vi "Timer_ResetInternal.vi"(11 "in TIMER":T1 {"Accumulated TIme" format="%13.5p"; "StartTime" format="%13.5p"}) -> (3 "out TIMER":T1 {"Accumulated TIme" format="%13.5p"; "StartTime" format="%13.5p"})   [LabVIEW 2019, in "Trajectory_Library.lvlib"]
doc: "THIS IS AN INTERNAL ROUTINE. DO NOT USE.\n \nReset the timer by setting the time to 0. Make the timer startTime the current time so new requests will be relative now\n\nInputs:\n - Timer -- The Timer data cluster\n\nOutputs:\n - Timer -- The modified Timer data cluster"
uses:
  Trajectory_Library.lvlib
  TIMER.ctl
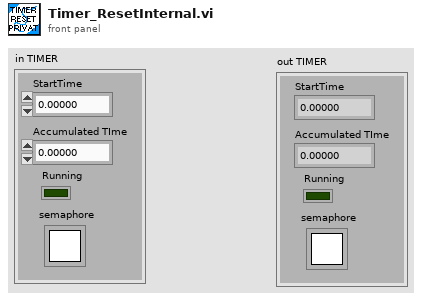
[diagram p1: front panel]
types:
  T1 = typedef "Trajectory_Library.lvlib/TIMER.ctl" = cluster{"StartTime":dbl, "Accumulated TIme":dbl, "Running":bool, "semaphore":T2}
  T2 = typedef "Semaphore RefNum" = refnum<k1>
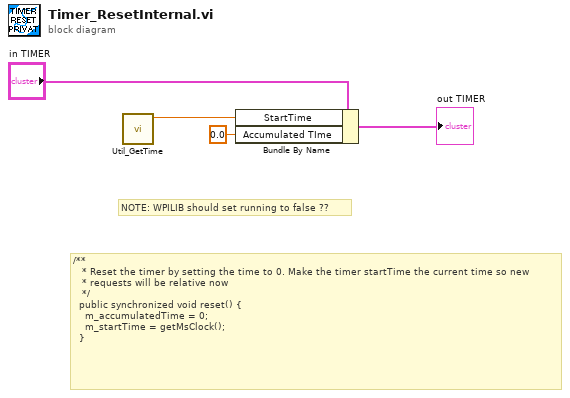
[diagram p0: block diagram]
diagram:
  # "NOTE: WPILIB should set running to false ??"
  # "/**\n   * Reset the timer by setting the time to 0. Make the timer startTime the current time so new\n   * requests will be relative now\n   */\n  public synchronized void reset() {\n    m_accumulatedTime = 0;\n    m_startTime = getMsClock();\n  }"
  n1 = call "Util_GetTime.vi"() -> ("FPGA_Time_Seconds"=w1:dbl)  [unwired: 10 in, 1 out]
  n2 = Bundle By Name(cluster="in TIMER", "StartTime"=w1, "Accumulated TIme"=0.0) -> (→"out TIMER":T1)
